vi "Create URI.vi"(8 "error in (no error)":errorcluster, 11 "uriString":string) -> (0 "error out":errorcluster, 3 ".NET Refnum out":refnum<k24>)   [LabVIEW 2018, in "LabVIEWHTTPClient_NET.lvlib" / "LabVIEWHTTPClient_NET.lvclass"]
uses:
  LabVIEWHTTPClient_NET.lvclass
  Types/HttpNet_error_enum.ctl
  LabVIEWHTTPClient_NET.lvlib
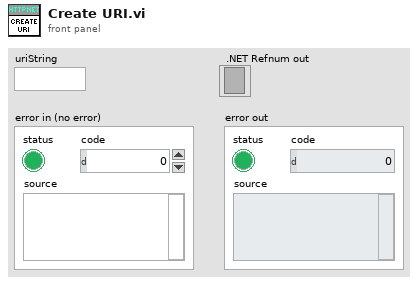
[diagram p1: front panel]
types:
  T1 = typedef "LabVIEWHTTPClient_NET.lvlib/HttpNet_error_enum.ctl" = enum16{"REST method is not available", "URL cannot be blank", "Output filepath cannot be empty", "Input filepath cannot be empty", "Internal .NET error %s", "Output filepath cannot be directory", "Download Task no longer exists"}
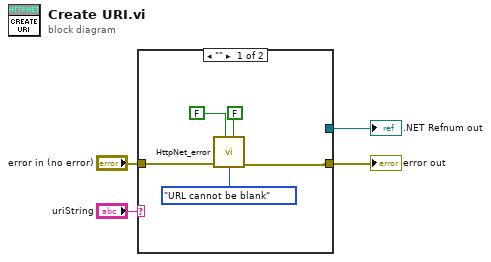
[diagram p0: block diagram]
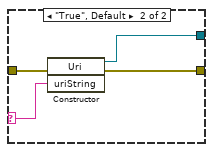
[diagram p2: hidden frame]
diagram:
  n1 = case shown="\"\"" "uriString" {
    selector: "uriString" -> [_ w13]
    tunnel: [w6 w12] -> w3
    tunnel: "error in (no error)" -> [w7 w11]
    tunnel: [_ w10] -> w1
    frame "" {
      n2 = call "HttpNet_error.vi"("ShowCallChain [T]"=FALSE, "OverrideExistingErrors [T]"=FALSE, "Error In"=w7, "Error"=HttpNet_error_enum."URL cannot be blank") -> ("Error Out"=w6:errorcluster)  [unwired: 7 in]
    }
    frame "True", Default {
      n3 = constructor class="Uri"(error in=w11, "uriString"=w13) -> (reference out=w10:refnum<k24>, error out=w12:errorcluster)  [unwired: 2 in, 2 out]
    }
  }
  "error out" <- w3
  ".NET Refnum out" <- w1
